vi "gbv.vi"() -> ()   [LabVIEW 2025]
panel:
  in  "ip":string
  out "host?":bool
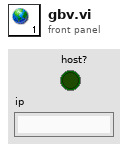
[diagram p1: front panel]
diagram:
